vi "Sliding Windows.vi"() -> ()   [LabVIEW 2020]
uses:
  <vilib>/regexp/Match Regular Expression.xnode
panel:
  out "Windowed Count":i32
  in  "Input":string="156\n153\n163\n168\n166\n164\n149\n187\n192\n194\n197\n199\n201\n210\n211\n196\n202\n203\n193\n199\n236\n240\n241\n251\n228\n226\n227\n256\n269\n270\n265\n271\n267\n271\n247\n254\n259\n258\n269\n270\n269\n267\n289\n290\n288\n309\n307\n299\n309\n326\n329\n332\n335\n338\n342\n333\n330\n332\n333\n334\n318\n317\n318\n316\n314\n315\n322\n327\n328\n331\n332\n338\n346\n341\n350\n334\n323\n322\n321\n325\n329\n342\n343\n353\n361\n355\n331\n329\n330\n319\n321\n322\n321\n322\n325\n316\n317\n322\n324\n331\n322\n323\n324\n325\n324\n336\n324\n335\n336\n337\n335\n336\n339\n343\n348\n353\n351\n349\n339\n341\n327\n322\n325\n298\n299\n306\n307\n321\n317\n314\n313\n316\n328\n325\n330\n331\n332\n339\n340\n348\n352\n354\n350\n374\n364\n370\n371\n379\n381\n380\n..."
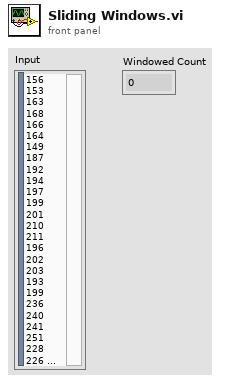
[diagram p1: front panel]
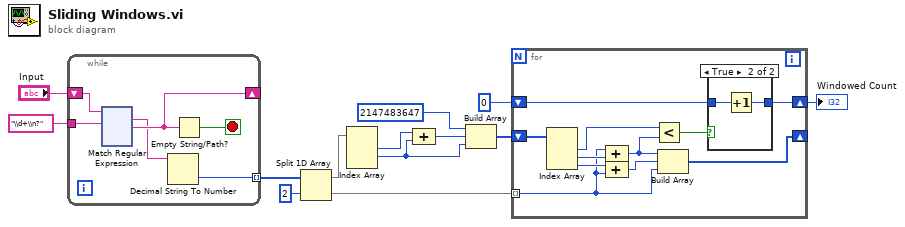
[diagram p0: block diagram]
diagram:
  n1 = while {
    shift-right: [w17] -> _
    shift-left: "Input" -> [w15]
    tunnel: "\\d+\\n?" -> [w19]
    tunnel: [w14] -> w11 mode=indexing
    stop <- w18 stop-if-true
    n2 = xnode "Match Regular Expression"("input string"=w15, "regular expression"=w19) -> ("whole match"=w16:string, "after match"=w17:string)  [unwired: 4 in, 3 out]
    n3 = Decimal String To Number(string=w16) -> (number=w14:i32)  [unwired: 2 in, 1 out]
    n4 = Empty String/Path?(string/path=w17) -> (empty?=w18:bool)
  }
  n5 = Split 1D Array(array=w11, index=2) -> (first subarray=w9:i32[], second subarray=w4:i32[])
  n6 = Index Array(array=w9) -> (element #1=w8:i32, element #2=w2:i32)  [unwired: 3 in, 1 out]
  n7 = Compound Arithmetic op=ADD(w8, w2) -> (w6:i32)
  n8 = Build Array(2147483647, w6, w2) -> (w5:i32[])
  n9 = for {
    shift-right: [w139] -> _
    shift-left: w5 -> [w144]
    tunnel: w4 -> [w140] mode=indexing
    shift-right: [w134] -> w1
    shift-left: 0 -> [w135]
    n10 = Index Array(array=w144) -> (element #1=w137:i32, element #2=w142:i32, element #3=w143:i32)  [unwired: 3 in]
    n11 = Compound Arithmetic op=ADD(w140, w142) -> (w138:i32)
    n12 = Compound Arithmetic op=ADD(w143, w140) -> (w141:i32)
    n13 = Less?(x=w137, y=w138) -> (x < y?=w136:bool)
    n14 = Build Array(w138, w141, w140) -> (w139:i32[])
    n15 = case shown="True" w136 {
      tunnel: w135 -> [w145 w147]
      tunnel: [w145 w146] -> w134
      frame False {
      }
      frame True {
        n16 = Increment(x=w147) -> (x+1=w146:i32)
      }
    }
  }
  "Windowed Count" <- w1
